vi "Parse Core.vi"(0 "Vector Path in":refnum<class "Vector Path.lvclass">, 5 "Config Row":string[](array[string]), 11 "error in (no error)":errorcluster) -> (4 "Vector Path out":refnum<class "Vector Path.lvclass">, 15 "error out":errorcluster)   [LabVIEW 2023, in "RFFixtureCharact.Public.lvlib" / "Vector Path.lvclass"]
uses:
  Public/Charact Result Accessor/Vector/Vector Charact Result Accessor.lvclass
  C:/rfcal/AuxTools/STSRFFixtureCharactUtility/Source/Code Modules/Fixture/Public/Charact Result Accessor/Base/Charact Result Accessor.lvclass
  C:/rfcal/AuxTools/STSRFFixtureCharactUtility/Source/Code Modules/Common/Result Accessor/Result Accessor.lvclass
  Common/Base Classes/Path/Path.lvclass/Path.ctl
  Common/Base Classes/Path/Properties/Read Interval.vi
  Public/Base Classes/Vector/Vector Path/Vector Path.lvclass
  Public/Base Classes/Vector/Vector Path/Vector Path.lvclass/Vector Path.ctl
  Public/Base Classes/Vector/Vector Abstract Path/Vector Abstract Path.lvclass
  C:/rfcal/AuxTools/STSRFFixtureCharactUtility/Source/Code Modules/Fixture/Public/Charact Result Accessor/Vector/Vector Charact Result Accessor.lvclass
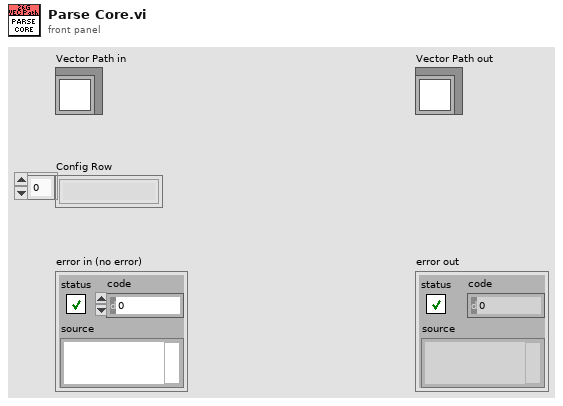
[diagram p1: front panel]
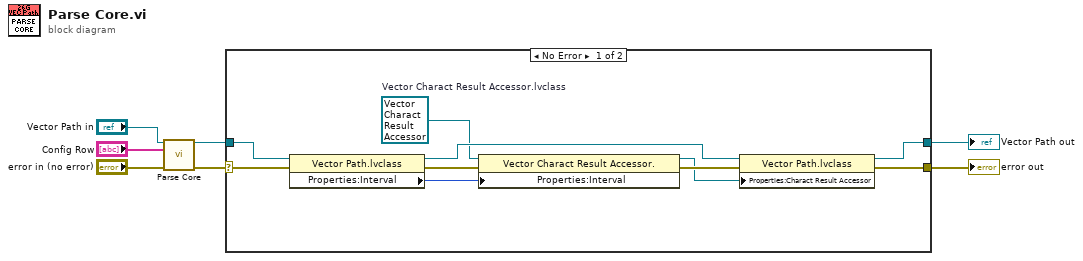
[diagram p0: block diagram]
diagram:
  n1 = call-parent "Parse Core.vi"("Vector Path in"="Vector Path in", "Config Row"="Config Row", "error in (no error)"="error in (no error)") -> ("Vector Path out"=w7:refnum<class "Vector Path.lvclass">, "error out"=w6:errorcluster)  [unwired: 11 in]
  n2 = case shown="No Error" w6 {
    selector: w6 -> [w8 w18]
    tunnel: w7 -> [w11 w19]
    tunnel: [w10 w18] -> w2
    tunnel: [w9 w19] -> w1
    frame No Error {
      w12 = refnum<class "Vector Charact Result Accessor.lvclass"> refnum  # Vector Charact Result Accessor.lvclass
      n3 = property class="Vector Path.lvclass"(reference=w11, error in=w8) -> (reference out=w14:refnum<class "Vector Path.lvclass">, error out=w16:errorcluster, "Properties:Interval"=w15:i32)
      n4 = property class="Vector Charact Result Accessor."(reference=w12, error in=w16, "Properties:Interval"=w15) -> (reference out=w13:refnum<class "Vector Charact Result Accessor.lvclass">, error out=w17:errorcluster)
      n5 = property class="Vector Path.lvclass"(reference=w14, error in=w17, "Properties:Charact Result Accessor"=w13) -> (reference out=w9:refnum<class "Vector Path.lvclass">, error out=w10:errorcluster)
    }
    frame Error {
    }
  }
  "error out" <- w2
  "Vector Path out" <- w1
